vi "Main.vi"   [LabVIEW 2023]
uses:
  TypeDefs/DataTypes/SystemStatus.ctl
types:
  T1 = typedef "SystemStatus.ctl" = cluster{"Bias Voltage":dbl, "SiPM Temperature":dbl[], "Slow Control User":string, "LXe":dbl}
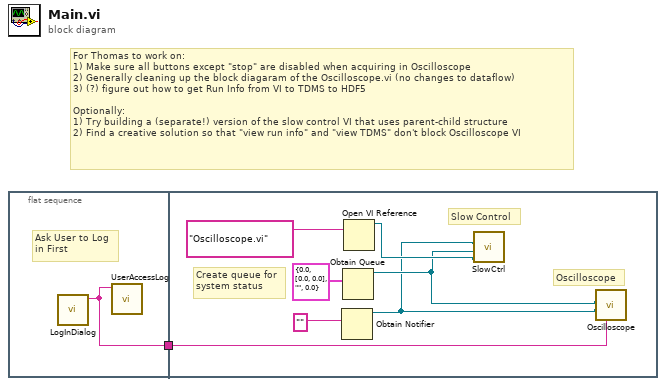
[diagram p0: block diagram]
diagram:
  # "For Thomas to work on:\n1) Make sure all buttons except \"stop\" are disabled when acquiring in Oscilloscope\n2) Generally cleaning up the block diagaram of the Oscilloscope.vi (no changes to dataflow)\n3) (?) figure out how to get Run Info from VI to TDMS to HDF5\n\nOptionally:\n1) Try building a (separate!) version of the slow control VI that uses parent-child structure\n2) Find a creative solution so that \"view run info\" and \"view TDMS\" don't block Oscilloscope VI"
  n1 = flat-sequence {
    tunnel: [w2] -> w1
    tunnel: w1 -> [w3]
    frame #0 {
      # "Ask User to Log\nin First"
      n2 = call "LogInDialog.vi"() -> ("Active User"=w2:string)  [unwired: 11 in]
      n3 = call "UserAccessLog.vi"("Active User"=w2) -> ()  [unwired: 11 in]
    }
    frame #1 {
      # "Create queue for\nsystem status"
      # "Oscilloscope"
      # "Slow Control"
      n4 = Obtain Notifier(notification data type="" ("String")) -> (notifier out=w4:refnum<notifier>)  [unwired: 3 in, 2 out]
      n5 = Obtain Queue(element data type=T1 {"Bias Voltage"=0.0, "SiPM Temperature"=[0.0, 0.0], "Slow Control User"="", "LXe"=0.0} ("System Status")) -> (queue out=w5:refnum<queue>)  [unwired: 4 in, 2 out]
      n6 = Open VI Reference(vi path="Oscilloscope.vi" ("String")) -> (vi reference=w6:refnum<vi>)  [unwired: 5 in, 1 out]
      n7 = call "SlowCtrl.vi"("Oscilloscope Ref"=w6, "queue in"=w5, "notifier in"=w4) -> ()  [unwired: 9 in]
      n8 = call "Oscilloscope.vi"("Slow Control User"=w3, "notifier in"=w4, "queue in"=w5) -> ()  [unwired: 9 in]
    }
  }
